vi "Get Device Outputs.vi"(8 "error in (no error)":errorcluster, 10 "Device Reference in":T8 format="%.0x", 11 "RT Data in":T1 {"Channels"."Voltage"."Ref"."Data Reference" format="%.0x"; "Channels"."Current"."Ref"."Data Reference" format="%.0x"; "Channels"."Read Volt"."Ref" format="%.0x"; "Channels"."Mode"."Ref" format="%.0x"}) -> (0 "error out":errorcluster, 2 "Device Ref out":T8 format="%.0x", 3 "RT Data out":T1 {"Channels"."Voltage"."Ref"."Data Reference" format="%.0x"; "Channels"."Current"."Ref"."Data Reference" format="%.0x"; "Channels"."Read Volt"."Ref" format="%.0x"; "Channels"."Mode"."Ref" format="%.0x"})   [LabVIEW 2011, in "Switch-DMM Custom Device.lvlib"]
uses:
  Switch-DMM Custom Device.lvlib
  <vilib>/NI Veristand/Custom Device API/Custom Device Item Ref.ctl
  Controls/RT Data.ctl
  Controls/Channels.ctl
  Controls/Single Channel.ctl
  <vilib>/NI Veristand/Custom Device API/Data Reference.ctl
  Controls/Block Channels.ctl
  <vilib>/NI Veristand/Custom Device API/Block Data Reference.ctl
  Controls/Communication.ctl
  Controls/Async Status.ctl
  Controls/Async State.ctl
  Controls/Async Command.ctl
  Controls/Async Events.ctl
  <vilib>/NI Veristand/Custom Device API/Custom Device Channel Type.ctl
  <vilib>/NI Veristand/Custom Device API/Data Access Type.ctl
  Controls/Globals.vi
  <vilib>/NI Veristand/Custom Device Tools/Custom Device Utility Library/NI VeriStand - Search for Item by Property.vi
  <vilib>/NI Veristand/Custom Device API/Custom Device API.lvlib
  <vilib>/NI Veristand/Custom Device Tools/Custom Device Utility Library/Custom Device Utility Library.lvlib
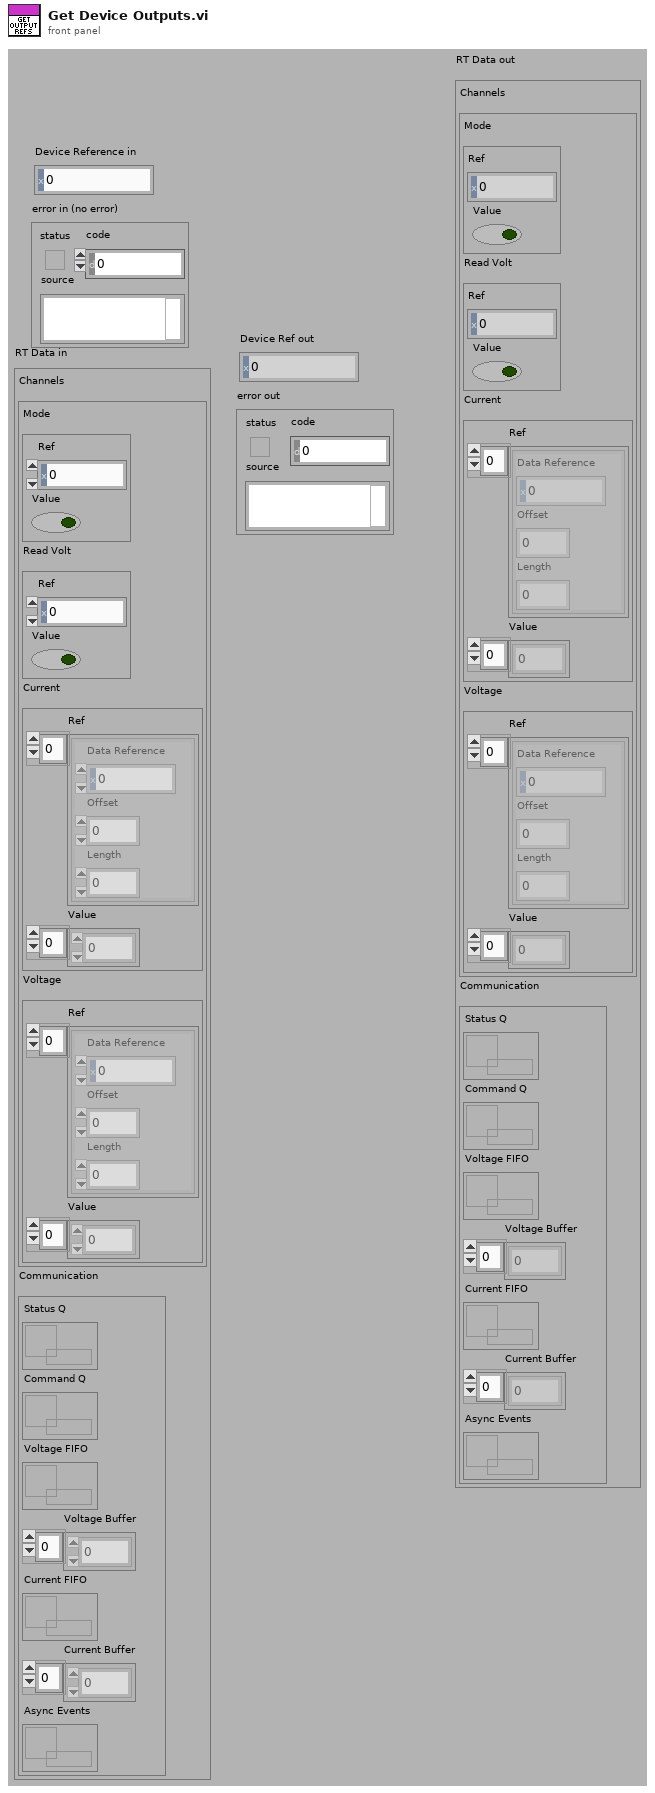
[diagram p1: front panel]
types:
  T1 = typedef "Switch-DMM Custom Device.lvlib/RT Data.ctl" = cluster{"Channels":T2, "Communication":T7}
  T2 = typedef "Switch-DMM Custom Device.lvlib/Channels.ctl" = cluster{"Mode":T3, "Read Volt":T3, "Current":T5, "Voltage":T5}
  T3 = typedef "Switch-DMM Custom Device.lvlib/Single Channel.ctl" = cluster{"Ref":T4, "Value":bool}
  T4 = typedef "Custom Device API.lvlib/Data Reference.ctl" = i32
  T5 = typedef "Switch-DMM Custom Device.lvlib/Block Channels.ctl" = cluster{"Ref":T6[], "Value":dbl[]}
  T6 = typedef "Custom Device API.lvlib/Block Data Reference.ctl" = cluster{"Data Reference":T4, "Offset":i32, "Length":i32}
  T7 = typedef "Switch-DMM Custom Device.lvlib/Communication.ctl" = cluster{"Status Q":refnum<queue>, "Command Q":refnum<queue>, "Voltage FIFO":refnum<k33>, "Voltage Buffer":dbl[], "Current FIFO":refnum<k33>, "Current Buffer":dbl[], "Async Events":refnum<queue>}
  T8 = typedef "Custom Device API.lvlib/Custom Device Item Ref.ctl" = u64
  T9 = typedef "Custom Device API.lvlib/Custom Device Channel Type.ctl" = enum16{"Input", "Output"}
  T10 = typedef "Custom Device API.lvlib/Data Access Type.ctl" = enum16{"Read", "Write"}
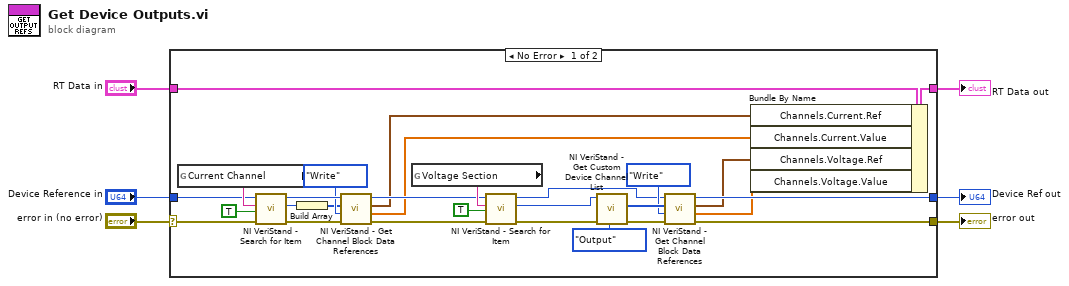
[diagram p0: block diagram]
diagram:
  n1 = case shown="No Error" "error in (no error)" {
    selector: "error in (no error)" -> [w27 w36]
    tunnel: [w34 w37] -> w6
    tunnel: [w30 w36] -> w5
    tunnel: "Device Reference in" -> [w26 w37]
    tunnel: "RT Data in" -> [w19 w35]
    tunnel: [w18 w35] -> w1
    frame No Error {
      n2 = global read "Globals.vi" "Current Channel"() -> (w28:string)
      n3 = call-poly <vilib>:"NI VeriStand - Search for Item.vi"("error in"=w27, "Property Value"=TRUE, "Property Name"=w28, "Section Ref in"=w26) -> ("error out"=w14:errorcluster, "Item Ref"=w11:T8, "Section Ref out"=w13:T8)  [unwired: 4 in, 1 out]
      n4 = Build Array(w11) -> (w10:T8[])
      n5 = call <vilib>:"NI VeriStand - Get Channel Block Data References.vi"("error in (no error)"=w14, "Access"=Data_Access_Type."Write", "Channel Refs"=w10, "Device Ref in"=w13) -> ("error out"=w15:errorcluster, "Values Array"=w7:dbl[], "Block Data Refs"=w8:T6[], "Device Ref out"=w9:T8)  [unwired: 4 in]
      n6 = global read "Globals.vi" "Voltage Section"() -> (w25:string)
      n7 = call-poly <vilib>:"NI VeriStand - Search for Item.vi"("error in"=w15, "Property Value"=TRUE, "Property Name"=w25, "Section Ref in"=w9) -> ("error out"=w22:errorcluster, "Item Ref"=w23:T8, "Section Ref out"=w20:T8)  [unwired: 4 in, 1 out]
      n8 = call <vilib>:"NI VeriStand - Get Custom Device Channel List.vi"("Channel Type"=Custom_Device_Channel_Type."Output", "error in (no error)"=w22, "Device Ref in"=w23) -> ("error out"=w31:errorcluster, "Specified Channel Ref List"=w33:T8[])  [unwired: 7 out]
      n9 = call <vilib>:"NI VeriStand - Get Channel Block Data References.vi"("error in (no error)"=w31, "Access"=Data_Access_Type."Write", "Channel Refs"=w33, "Device Ref in"=w20) -> ("error out"=w30:errorcluster, "Values Array"=w16:dbl[], "Block Data Refs"=w17:T6[], "Device Ref out"=w34:T8)  [unwired: 4 in]
      n10 = Bundle By Name(cluster=w19, "Channels.Current.Ref"=w8, "Channels.Current.Value"=w7, "Channels.Voltage.Ref"=w17, "Channels.Voltage.Value"=w16) -> (w18:T1)
    }
    frame Error {
    }
  }
  "Device Ref out" <- w6
  "error out" <- w5
  "RT Data out" <- w1
